vi "Queue New Plugin Command.vi"(8 "error in (no error)":errorcluster, 10 "New Plugin":T1, 11 "CIFPluginManager in":refnum<class "CIFPluginManager.lvclass">) -> (0 "error out":errorcluster)   [LabVIEW 2021, in "CIFPluginManager.lvclass"]
uses:
  CIFPluginManager.lvclass
  typedef/Plugin Load Command.ctl
  typedef/Loader Type.ctl
  CIFPluginManager.lvclass/CIFPluginManager.ctl
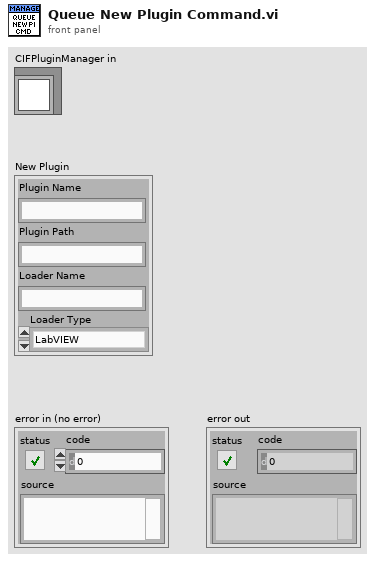
[diagram p1: front panel]
types:
  T1 = typedef "CIFPluginManager.lvclass/Plugin Load Command.ctl" = cluster{"Plugin Name":string, "Plugin Path":string, "Loader Name":string, "Loader Type":T2}
  T2 = typedef "CIFPluginManager.lvclass/Loader Type.ctl" = enum16{"LabVIEW"}
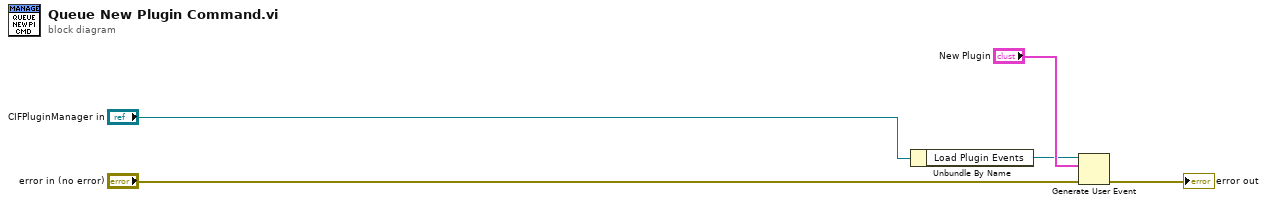
[diagram p0: block diagram]
diagram:
  n1 = Unbundle By Name("CIFPluginManager in") -> ("Load Plugin Events"=w2:refnum<user-event>)
  n2 = Generate User Event(user event=w2, event data cluster="New Plugin", error in="error in (no error)") -> (error out=→"error out":errorcluster)  [unwired: 1 in, 1 out]
